vi "tipdefinition.vi"(0 "#points":i32, 5 "radius of curvature":dbl min=-0.0 max=1000.0 format="%.2f", 9 "tipangle":dbl=1.0 min=1.0 max=89.0 format="%.2f", 11 "offset":i32=1) -> (6 "output":dbl[](array[numeric]) format="%.2f")   [LabVIEW 2017]
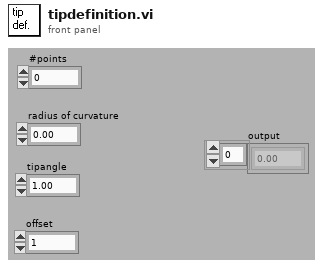
[diagram p1: front panel]
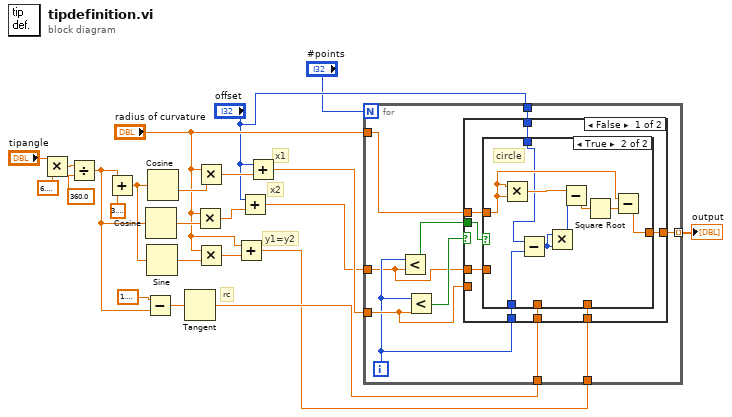
[diagram p0: block diagram]
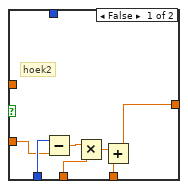
[diagram p2: hidden frame]
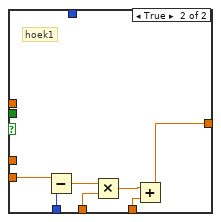
[diagram p3: hidden frame]
diagram:
  # "rc"
  # "y1=y2"
  # "x2"
  # "x1"
  n1 = Multiply(x="tipangle", y=6.283185307179586) -> (x*y=w21:dbl)
  n2 = Divide(x=w21, y=360.0) -> (x/y=w10:dbl)
  n3 = Add(x=w10, y=3.141592653589793) -> (x+y=w14:dbl)
  n4 = Subtract(x=1.5707963267948966, y=w10) -> (x-y=w9:dbl)
  n5 = Cosine(x=w10) -> (cos(x)=w17:dbl)
  n6 = Sine(x=w14) -> (sin(x)=w13:dbl)
  n7 = Cosine(x=w14) -> (cos(x)=w18:dbl)
  n8 = Tangent(1:w9) -> (0:w6:dbl)
  n9 = Multiply(x="radius of curvature", y=w17) -> (x*y=w16:dbl)
  n10 = Multiply(x="radius of curvature", y=w18) -> (x*y=w15:dbl)
  n11 = Multiply(x="radius of curvature", y=w13) -> (x*y=w12:dbl)
  n12 = Add(x="radius of curvature", y=w12) -> (x+y=w5:dbl)
  n13 = Add(x="offset", y=w16) -> (x+y=w7:dbl)
  n14 = Add(x="offset", y=w15) -> (x+y=w8:dbl)
  n15 = for {
    N: "#points" -> [_]
    tunnel: w8 -> [w32]
    tunnel: w7 -> [w29]
    tunnel: w6 -> [w30]
    tunnel: w5 -> [w28]
    tunnel: [w27] -> w3 mode=indexing
    tunnel: "radius of curvature" -> [w25]
    tunnel: "offset" -> [w24]
    i -> [w31]
    n16 = Less?(x=w31, y=w29) -> (x < y?=w26:bool)
    n17 = Less?(x=w31, y=w32) -> (x < y?=w33:bool)
    n18 = case shown="False" w33 {
      tunnel: w32 -> [_ w64]
      tunnel: w31 -> [w40 w63]
      tunnel: w30 -> [w39 w61]
      tunnel: [w37 w58] -> w27
      tunnel: w29 -> [w41 _]
      tunnel: w28 -> [w38 w60]
      tunnel: w26 -> [w36 _]
      tunnel: w25 -> [w35 _]
      tunnel: w24 -> [w34 _]
      frame False {
        n19 = case shown="True" w36 {
          tunnel: w41 -> [w47 _]
          tunnel: w40 -> [w48 w57]
          tunnel: w39 -> [w45 _]
          tunnel: w38 -> [w43 _]
          tunnel: [w42 w50] -> w37
          tunnel: w35 -> [_ w51]
          tunnel: w34 -> [_ w49]
          frame False {
            # "hoek2"
            n20 = Subtract(x=w48, y=w47) -> (x-y=w46:dbl)
            n21 = Multiply(x=w46, y=w45) -> (x*y=w44:dbl)
            n22 = Add(x=w44, y=w43) -> (x+y=w42:dbl)
          }
          frame True {
            # "circle"
            n23 = Multiply(x=w51, y=w51) -> (x*y=w56:dbl)
            n24 = Subtract(x=w49, y=w57) -> (x-y=w55:i32)
            n25 = Multiply(x=w55, y=w55) -> (x*y=w54:i32)
            n26 = Subtract(x=w56, y=w54) -> (x-y=w53:dbl)
            n27 = Square Root(x=w53) -> (sqrt(x)=w52:dbl)
            n28 = Subtract(x=w51, y=w52) -> (x-y=w50:dbl)
          }
        }
      }
      frame True {
        # "hoek1"
        n29 = Subtract(x=w64, y=w63) -> (x-y=w62:dbl)
        n30 = Multiply(x=w62, y=w61) -> (x*y=w59:dbl)
        n31 = Add(x=w59, y=w60) -> (x+y=w58:dbl)
      }
    }
  }
  "output" <- w3
